vi "AnalogSetEnabled.vi"(0 "error in (no error)":errorcluster, 1 "SetEnabled":bool, 2 "index":i32, 3 "Device In":i32) -> (7 "error out":errorcluster, 10 "Device Out":i32)   [LabVIEW 2013]
uses:
  phidget21.dll
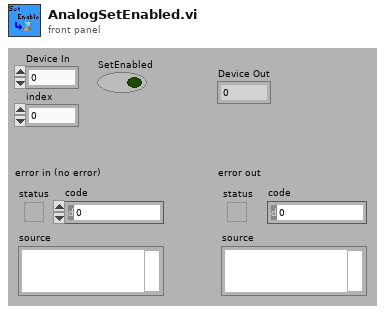
[diagram p1: front panel]
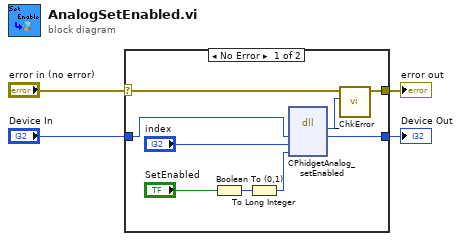
[diagram p0: block diagram]
diagram:
  n1 = case shown="No Error" "error in (no error)" {
    selector: "error in (no error)" -> [w9 w15]
    tunnel: [w8 w15] -> w3
    tunnel: "Device In" -> [w12 w14]
    tunnel: [w11 w14] -> w1
    frame No Error {
      n2 = Boolean To (0,1)(Boolean="SetEnabled") -> (0, 1=w7:i16)
      n3 = To Long Integer(number=w7) -> (32bit integer=w6:i32)
      n4 = dll-call lib="phidget21.*" fn="CPhidgetAnalog_setEnabled"("phid"=w12, "index"="index", "SetEnabled"=w6) -> (w10:i32, "phid"=w11:i32)  [unwired: 5 in, 2 out]
      n5 = call "_ChkError.vi"("Return Code"=w10, "error in (no error)"=w9) -> ("error out"=w8:errorcluster)  [unwired: 9 in]
    }
    frame Error {
    }
  }
  "error out" <- w3
  "Device Out" <- w1
